vi "CryoServer Read Telemetry.vi"(8 "error in (no error)":errorcluster, 10 "timeout ms (500)":i32=1000, 11 "CryoServer in":refnum<class "CryoServer.lvclass">) -> (0 "error out":errorcluster, 1 "Values":dbl[](array[numeric]), 2 "Ch Names":string[](array[string]), 3 "CryoServer out":refnum<class "CryoServer.lvclass">, 4 "Timestamp":timestamp, 6 "Board":string)   [LabVIEW 2021, in "CryoServer.lvclass"]
uses:
  CryoServer.lvclass
  CryoServer.lvclass/CryoServer.ctl
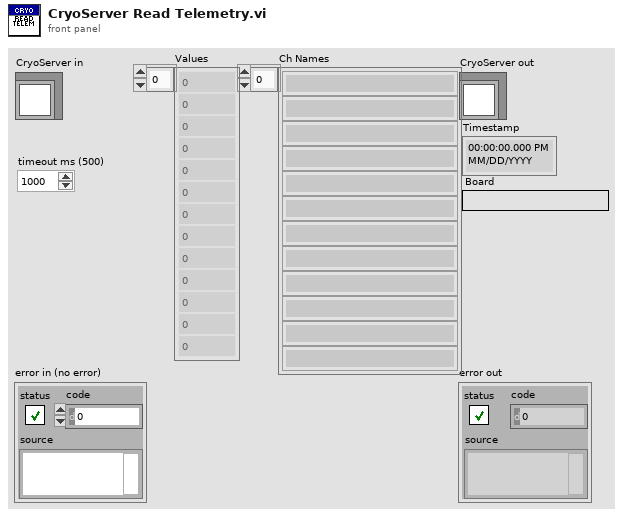
[diagram p1: front panel]
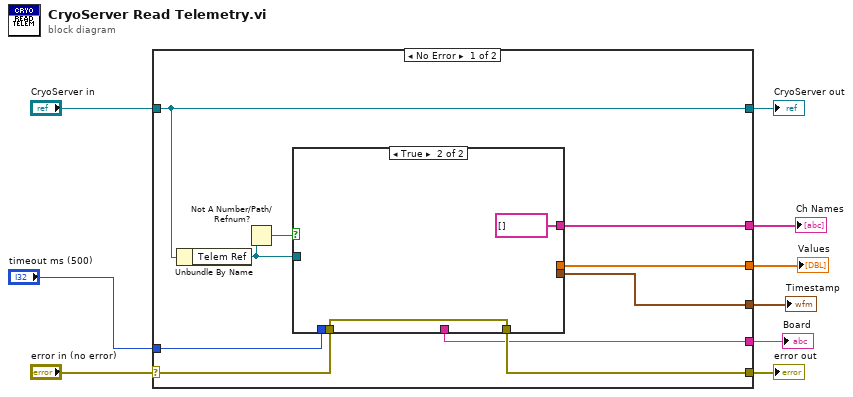
[diagram p0: block diagram]
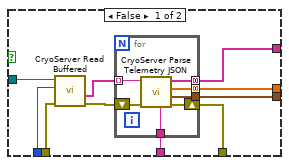
[diagram p2: hidden frame]
diagram:
  n1 = case shown="No Error" "error in (no error)" {
    selector: "error in (no error)" -> [w14 w40]
    tunnel: [w17 w40] -> w8
    tunnel: [w19 w39] -> w6
    tunnel: "CryoServer in" -> [w19 w39]
    tunnel: [w18 _] -> w5
    tunnel: [w16 _] -> w4
    tunnel: [w15 _] -> w3
    tunnel: [w12 _] -> w2
    tunnel: "timeout ms (500)" -> [w13 _]
    frame No Error {
      n2 = Unbundle By Name(w19) -> ("Telem Ref"=w10:refnum<k5>)
      n3 = Not A Number/Path/Refnum?(number/path/refnum=w10) -> (NaN/Path/Refnum?=w11:bool)
      n4 = case shown="True" w11 {
        tunnel: [w29 string[] [] ("Ch Names")] -> w18
        tunnel: [w28 w37] -> w17
        tunnel: [w27 _] -> w16
        tunnel: [w26 _] -> w15
        tunnel: w10 -> [w25 _]
        tunnel: w14 -> [w24 w37]
        tunnel: w13 -> [w23 _]
        tunnel: [w20 _] -> w12
        frame False {
          n5 = call "CryoServer Read Buffered.vi"("error in (no error)"=w24, "timeout ms (5000)"=w23, "connection ID"=w25) -> ("error out"=w22:errorcluster, "messages"=w21:string[])  [unwired: 5 in, 2 out]
          n6 = for {
            tunnel: [w36] -> w29 mode=concatenating
            tunnel: [w34] -> w27 mode=concatenating
            tunnel: [w33] -> w26
            shift-right: [w35] -> w28
            shift-left: w22 -> [w32]
            tunnel: w21 -> [w31] mode=indexing
            tunnel: [w30] -> w20
            n7 = call "CryoServer Parse Telemetry JSON.vi"("error in (no error)"=w32, "Telemetry String"=w31) -> ("error out"=w35:errorcluster, "Timestamp"=w33:timestamp, "Values"=w34:dbl[], "Ch Names"=w36:string[], "Board"=w30:string)  [unwired: 5 in]
          }
        }
        frame True {
        }
      }
    }
    frame Error {
    }
  }
  "error out" <- w8
  "CryoServer out" <- w6
  "Ch Names" <- w5
  "Values" <- w4
  "Timestamp" <- w3
  "Board" <- w2
